vi "fpga_MagnitudePhase (P Class).vi"(0 "re":fxp<+/-,32,6> format="%.29g", 1 "reset":bool, 5 "im":fxp<+/-,32,6> format="%.29g", 7 "Ch":fxp<+,5,5>=6.0, 9 "input valid":bool, 12 "ready for output":bool) -> (4 "rms magnitude":fxp<+,32,6> format="%.28g", 6 "phase":fxp<+/-,32,2> format="%.31g", 10 "output valid":bool, 14 "ready for input":bool)   [LabVIEW 2013, in "NI_EP_PMU_FPGA.lvlib"]
uses:
  <vilib>/addons/Electrical Power/PMU/NI_EP_PMU_FPGA.lvlib
  <vilib>/rvi/FXPMathLib/FxpRectToPolar/subVIs/nifxpmath_RectToPolar_SimConfig.ctl
  <vilib>/rvi/Emulation/niFpgaSctlEmulationGetInTimedLoop.vi
  <vilib>/rvi/eio/common/nirviEmuReportErrorAndStop.vi
  <vilib>/rvi/DataTransferAndStorage/Container/Common/niFpgaContainerSetEmuInfo.vi
  <vilib>/rvi/DataTransferAndStorage/Container/Common/niFpgaContainerGetUniqueNameForEmu.vi
  <vilib>/rvi/FXPMathLib/FxpRectToPolar/simVIs/DllFxpRectToPolarTemp_sub.vi
  <vilib>/rvi/Memory/Memory_Emulation/nirvimemoryEmulation.vi
  <vilib>/rvi/Memory/Memory_Emulation/nirvimemoryFastEmulation.vi
  <vilib>/rvi/Memory/Memory_Emulation/nirvimemoryEmulationManagerCache_ReleaseExclusive.vi
  <vilib>/rvi/Memory/Memory_Emulation/niFpgaMemoryEmulationValidateCache.vi
  <vilib>/rvi/Memory/Memory_Emulation/nirvimemoryEmulationManagerCache_MakeExclusive.vi
  <vilib>/rvi/Memory/Memory_Emulation/niFpgaMemoryEmulationCacheClearOnFirstRun.vi
  <vilib>/rvi/Memory/Memory_Emulation/nirvimemoryEmulationManagerCache_InsertValue.vi
  <vilib>/Utility/error.llb/Clear Errors.vi
  <vilib>/rvi/Memory/Memory_Emulation/nirvimemoryEmulationManagerCache_GetValue.vi
  <vilib>/rvi/LocalResourceManager/LocalResourceManager.xnode
  <vilib>/rvi/FXPMathLib/FxpRectToPolar/XNode/nifxpmath_RectToPolar.xnode
  <vilib>/rvi/FXPMathLib/basic elements/FxpDiscreteDelay/XNode/nifxpmath_DiscreteDelay.xnode
  <vilib>/rvi/DataTransferAndStorage/Container/XNode/niFpgaContainer.xnode
  <vilib>/rvi/FXPMathLib/FxpAdd/XNode/nifxpmath_Add.xnode
  <vilib>/addons/Electrical Power/PQ/Resampling/NI_EP_Resample_FPGA.lvlib
  <vilib>/rvi/FXPMathLib/sim/FxpSim.dll
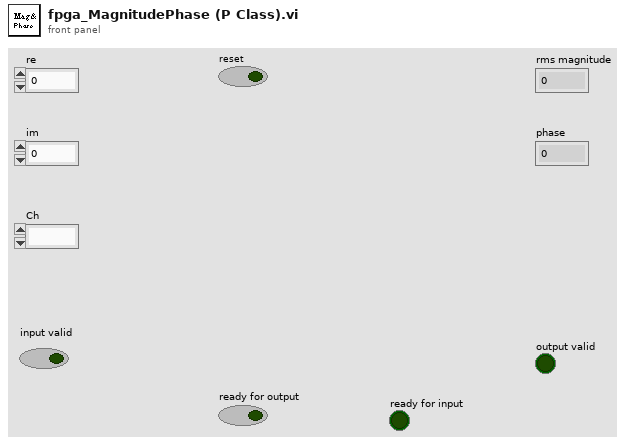
[diagram p1: front panel]
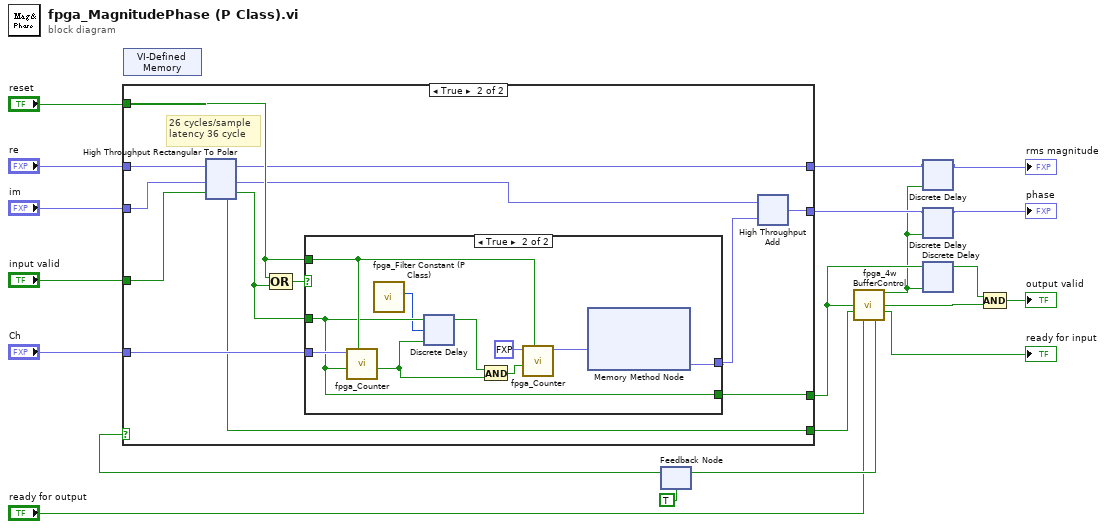
[diagram p0: block diagram]
diagram:
  n1 = xnode "VI-Defined Memory"() -> ()  [unwired: 1 out]
  n2 = feedback #1(TRUE ("logic enable")) -> (w16:bool)
  n3 = case shown="True" w16 {
    tunnel: "input valid" -> [_ w29]
    tunnel: "reset" -> [_ w28]
    tunnel: "Ch" -> [_ w27]
    tunnel: "re" -> [_ w31]
    tunnel: "im" -> [_ w30]
    tunnel: [_ w24] -> w7
    tunnel: [_ w25] -> w8
    tunnel: [_ w26] -> w5
    tunnel: [_ w21] -> w3
    frame False {
    }
    frame True {
      # "26 cycles/sample\nlatency 36 cycle"
      n4 = xnode "High Throughput Rectangular To Polar"("x"=w31, "y"=w30, "input valid"=w29) -> ("magnitude"=w21:fxp<+,32,6>, "phase (pi)"=w22:fxp<+/-,32,2>, "output valid"=w32:bool, "ready for input"=w25:bool)  [unwired: 1 in]
      n5 = Compound Arithmetic op=OR(w28, w32) -> (w33:bool)
      n6 = case shown="True" w33 {
        tunnel: [_ w43] -> w23
        tunnel: [_ w36] -> w24
        tunnel: w27 -> [_ w42]
        tunnel: w32 -> [_ w36]
        tunnel: w28 -> [_ w41]
        frame False {
        }
        frame True {
          n7 = call <vilib>:"fpga_Counter.vi"("reset"=w41, "Input Valid?"=w36, "upper limit"=w42) -> ("Multichannel Valid?"=w37:bool)  [unwired: 7 in, 1 out]
          n8 = call <vilib>:"fpga_Filter Constant (P Class).vi"() -> ("LP2 delay"=w34:u8)  [unwired: 8 in, 3 out]
          n9 = xnode ("Discrete Delay")("D"=w36, "n-1[0..23]"=w34, "enable"=w37) -> ("Q"=w35:bool)
          n10 = And(x=w35, y=w37) -> (x .and. y?=w40:bool)
          n11 = call <vilib>:"fpga_Counter.vi"("reset"=w41, "Input Valid?"=w40, "upper limit"=fxp<+,5,5> 25.0 ("#ch")) -> ("count"=w39:fxp<+,5,5>)  [unwired: 7 in, 1 out]
          n12 = xnode ("Memory Method Node")("Address"=w39) -> ("Data"=w43:fxp<+/-,32,2>)  [unwired: 1 in, 1 out]
        }
      }
      n13 = xnode ("High Throughput Add")("x"=w22, "y"=w23) -> ("x+y"=w26:fxp<+/-,32,2>)
    }
  }
  n14 = call <vilib>:"fpga_4w BufferControl.vi"("DR"=w7, "RFI"=w8, "RFO"="ready for output") -> ("buff enable"=w2:bool, "output valid"=w18:bool, "ready for input"=→"ready for input":bool, "logic enable"=w17:bool)  [unwired: 9 in]
  n15 = feedback-in #1(w17) -> ()
  n16 = xnode ("Discrete Delay")("D"=w3, "enable"=w2) -> ("Q"=→"rms magnitude":fxp<+,32,6>)
  n17 = xnode ("Discrete Delay")("D"=w5, "enable"=w2) -> ("Q"=→"phase":fxp<+/-,32,2>)
  n18 = xnode ("Discrete Delay")("D"=w7, "enable"=w2) -> ("Q"=w6:bool)
  n19 = Compound Arithmetic op=AND(w6, w18) -> (→"output valid":bool)
